vi "断点管理器.vi"() -> ()   [LabVIEW 2010]
panel:
  in  "停止":bool
  in  "y":dbl
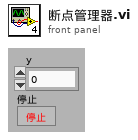
[diagram p1: front panel]
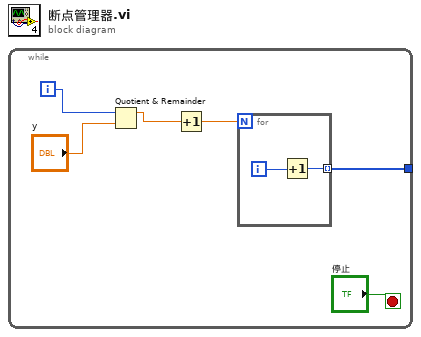
[diagram p0: block diagram]
diagram:
  n1 = while {
    tunnel: [w2] -> _
    i -> [w6]
    stop <- "停止" stop-if-true
    n2 = Quotient & Remainder(x=w6, y="y") -> (x-y*floor(x/y)=w4:dbl)  [unwired: 1 out]
    n3 = Increment(x=w4) -> (x+1=w3:dbl)
    n4 = for {
      N: w3 -> [_]
      tunnel: [w7] -> w2 mode=indexing
      i -> [w8]
      n5 = Increment(x=w8) -> (x+1=w7:i32)
    }
  }
